vi "FTW-JSON-Core-Serialize.vi"(0 "JSON Object":i64 format="%016x", 5 "Encoding Flags":i64 format="%016x", 11 "error in":errorcluster) -> (4 "JSON Object":i64 format="%016x", 6 "JSON String (UTF-8)":string, 15 "error out":errorcluster)   [LabVIEW 2014]
uses:
  error/FTW-ERR-ThrowGenericError.vi
  error/FTW-ERR-ThrowError.vi
  error/FTW-ERR-NoErrorConstant.vi
  string/FTW-STR-ReplaceWhitespace.vi
  error/FTW-ERR-CallChain.vi
panel:
  # "Inputs"
  # "Outputs"
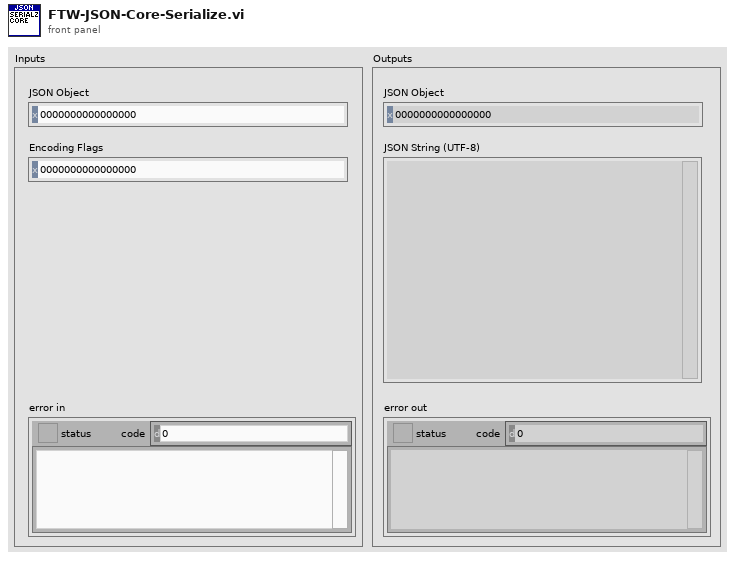
[diagram p1: front panel]
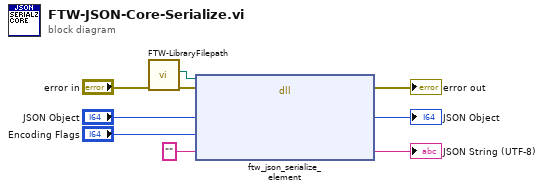
[diagram p0: block diagram]
diagram:
  n1 = call "FTW-LibraryFilepath.vi"("error in"="error in") -> ("error out"=w2:errorcluster, "Library Filepath"=w1:path)  [unwired: 8 in, 1 out]
  n2 = dll-call lib="?" fn="ftw_json_serialize_element"(path in=w1, error in=w2, "JSON Object Pointer"="JSON Object", "Flags"="Encoding Flags", "Serialized String"="") -> (error out=→"error out":errorcluster, "JSON Object Pointer"=→"JSON Object":i64, "Serialized String"=→"JSON String (UTF-8)":string)  [unwired: 3 in, 1 out]
